vi "Test_KEITHLEY2470.vi"(8 "error in (no error)":errorcluster) -> (0 "error out":errorcluster)   [LabVIEW 2019]
uses:
  Type Definition/handle_Para.ctl
panel:
  in  "VISA resource name out":refnum<visa-resource-name>
  in  "Source Mode  (0: Voltage)":u16(ring) items=["Voltage", "Current"]
  out "lt":u32
  out "Curr[A]":dbl format="%#_6p"
  out "Volt[V]":dbl format="%#_6p"
  in  "STOP":bool
  out "Waveform Chart":cluster{"data[0]":dbl, "data[1]":dbl}(graph)
  in  "READ":bool
  in  "Source Limit Level":dbl=0.01
  in  "Source Level":dbl
  in  "OFF":bool
  in  "ON":bool
  # "KEITHLEY"
  # "2470 SMU"
  # "LEVEL SET"
  # "OUTPUT"
  # "READ"
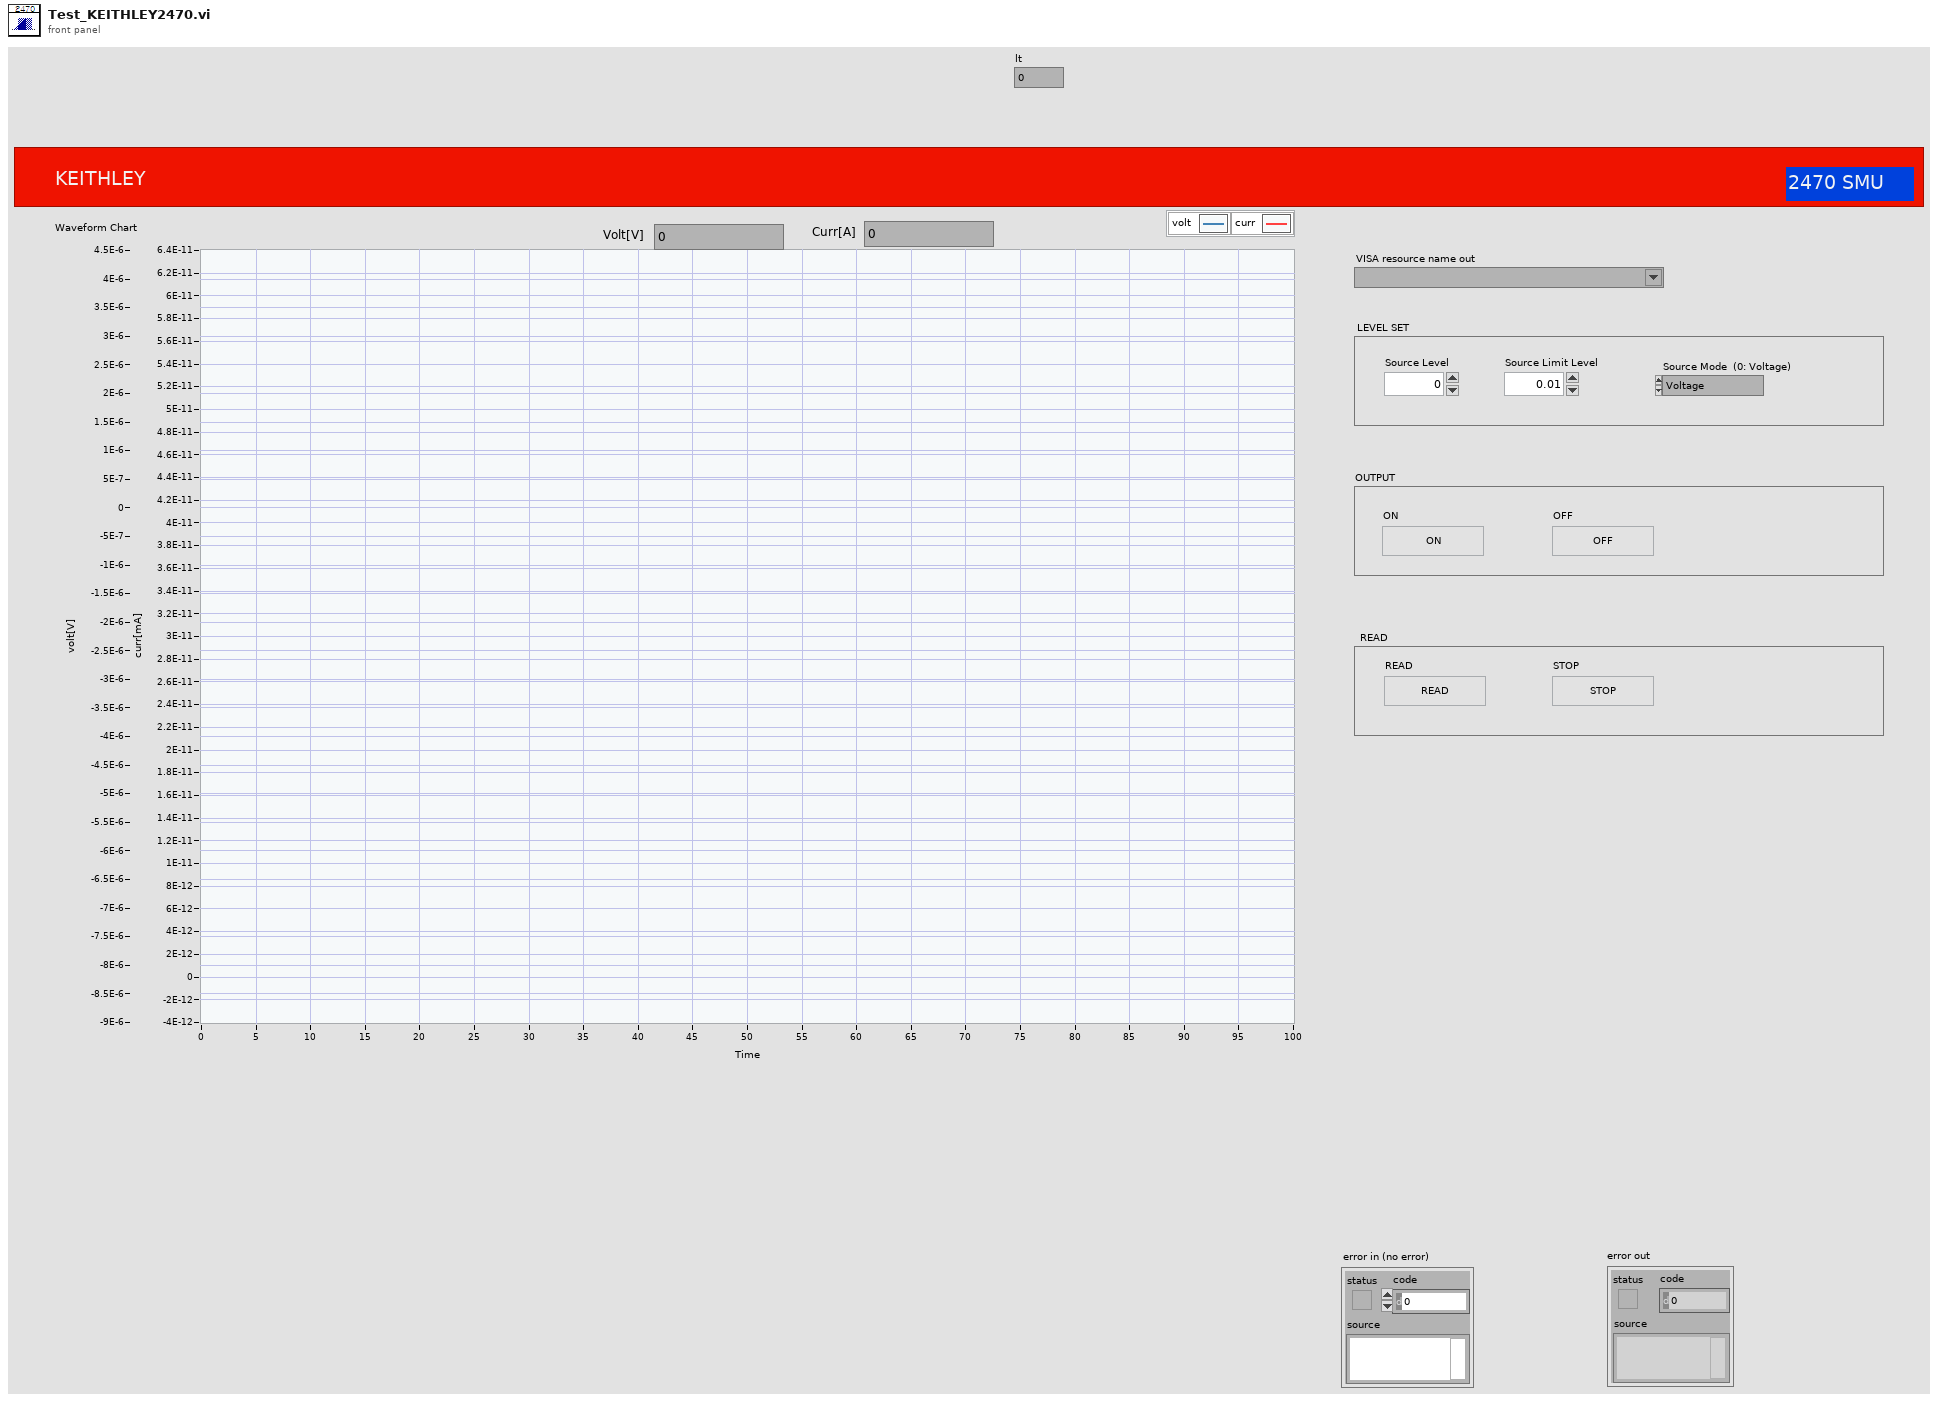
[diagram p1: front panel]
types:
  T1 = typedef "handle_Para.ctl" = cluster{"VISA resource name":refnum<visa-resource-name>, "Function (0: Volts) 1":u16, "Function (0: Volts) 2 ":u16, "Enable Auto Range (T:Enable)":bool, "Source Mode  (0: Voltage)":u16, "Source Level (0)":dbl, "Source Limit Level (0.1)":dbl}
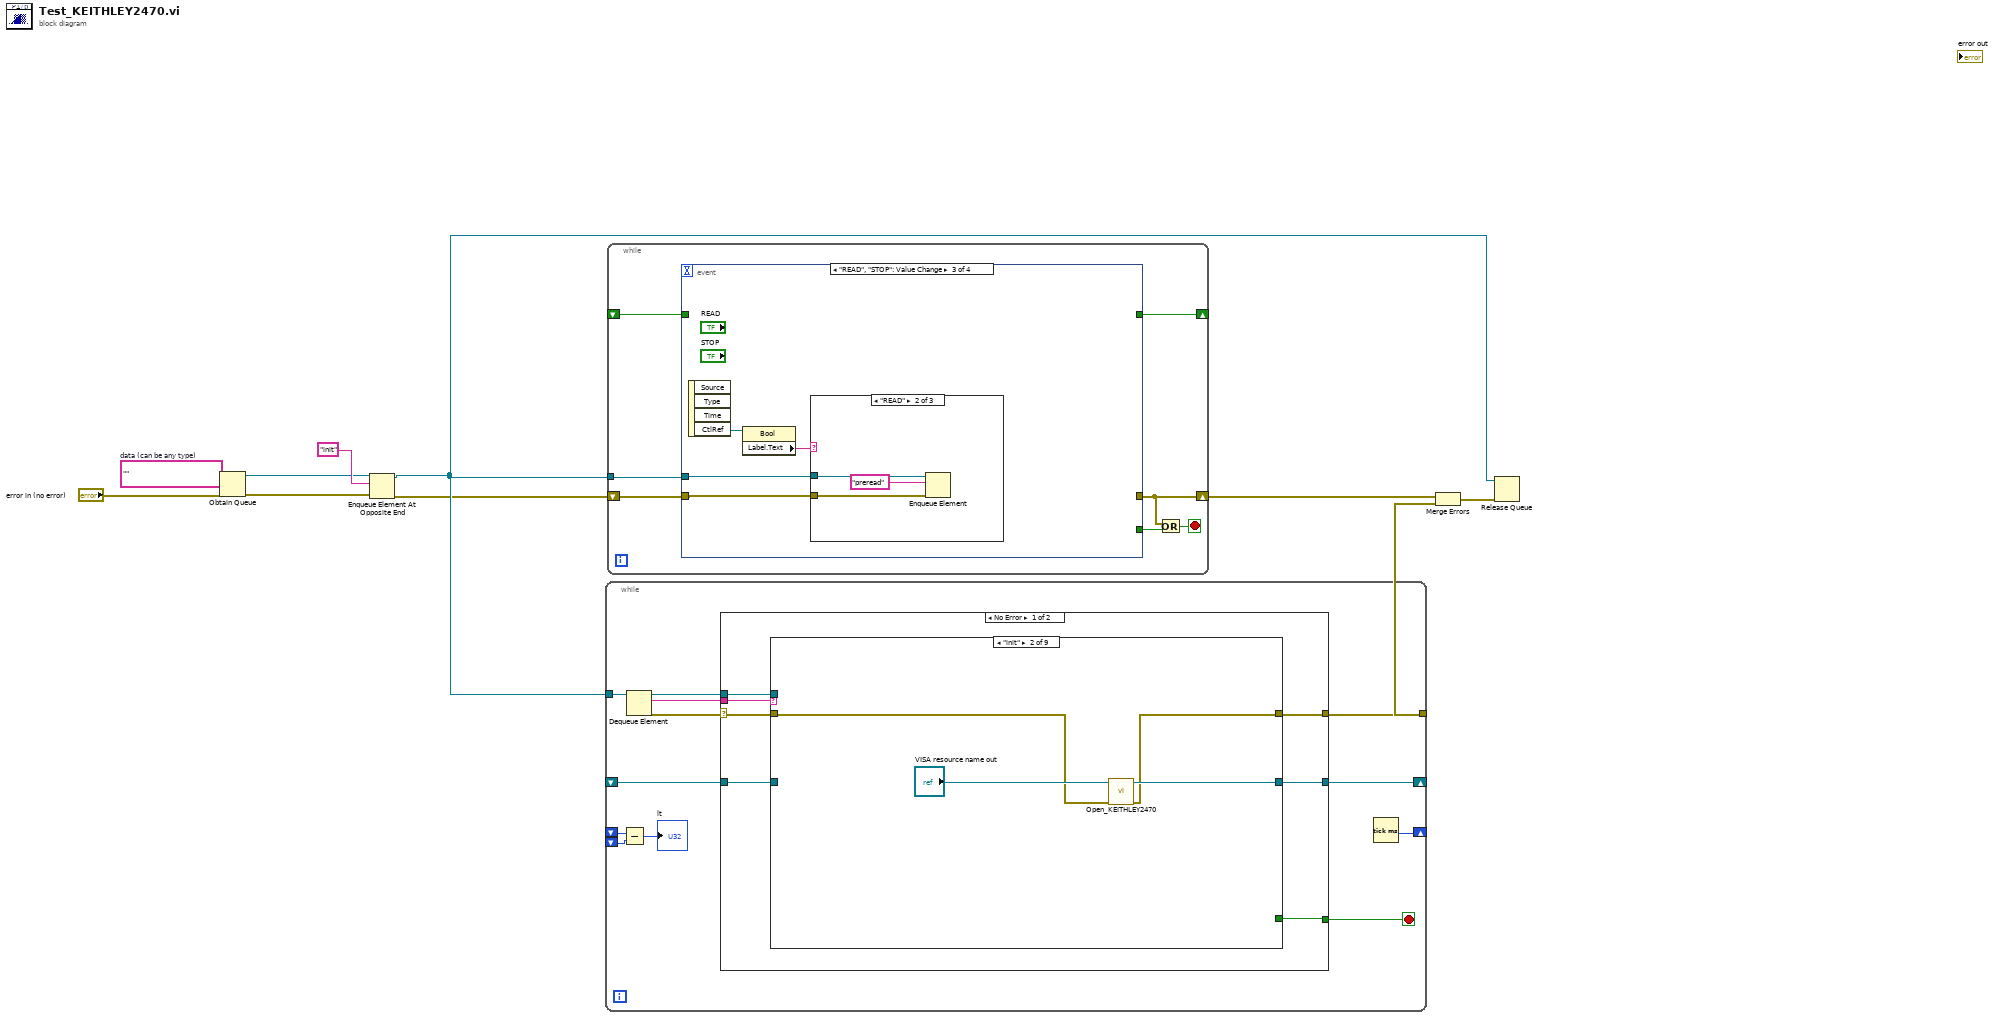
[diagram p0: block diagram]
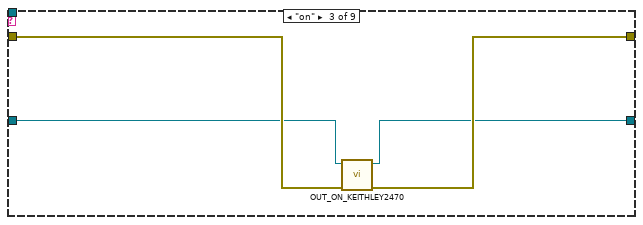
[diagram p3: hidden frame]
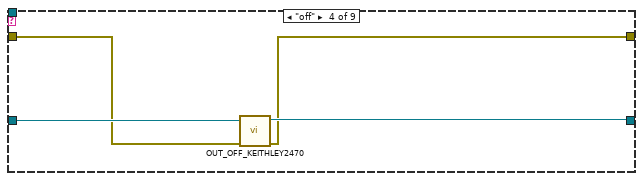
[diagram p4: hidden frame]
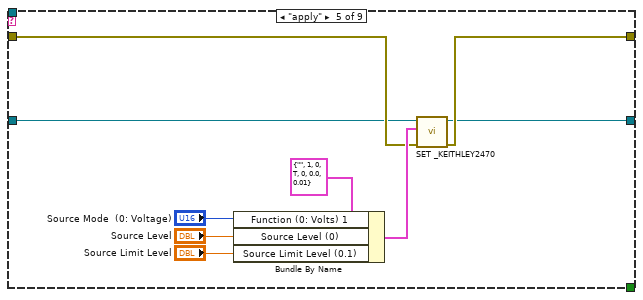
[diagram p5: hidden frame]
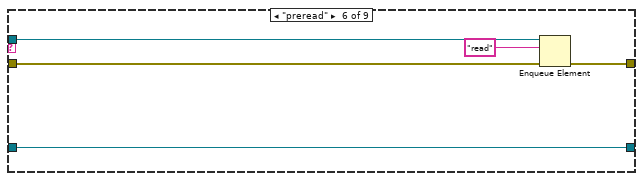
[diagram p6: hidden frame]
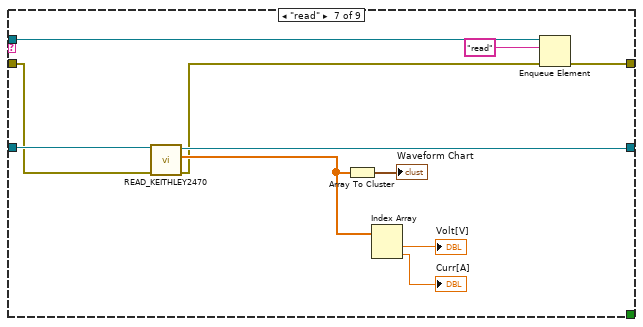
[diagram p7: hidden frame]
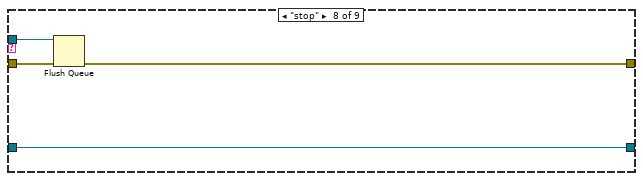
[diagram p8: hidden frame]
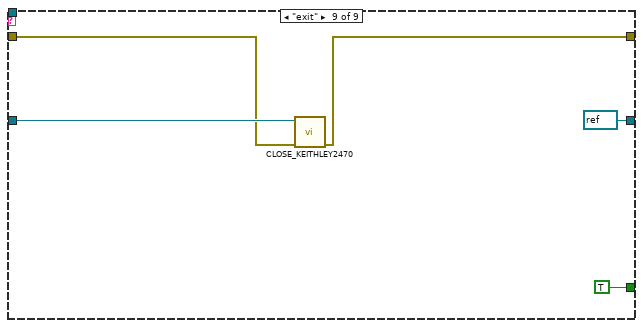
[diagram p9: hidden frame]
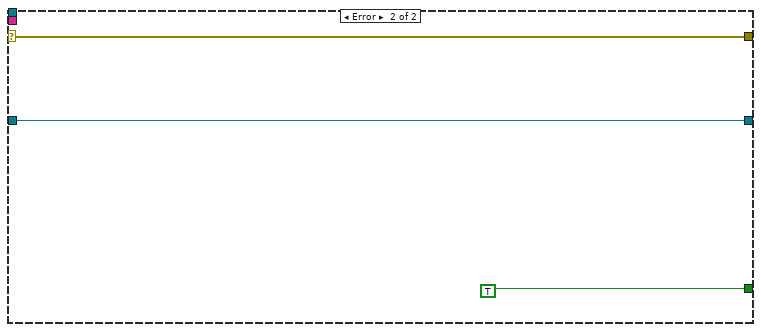
[diagram p10: hidden frame]
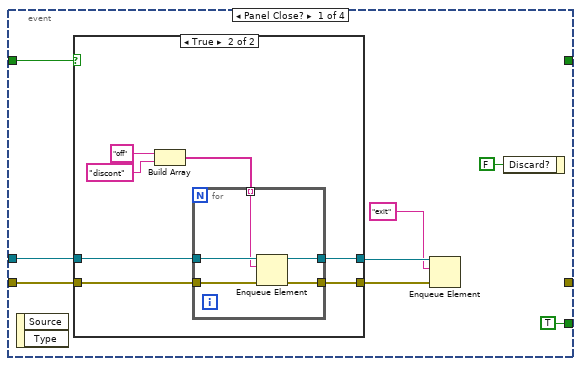
[diagram p11: hidden frame]
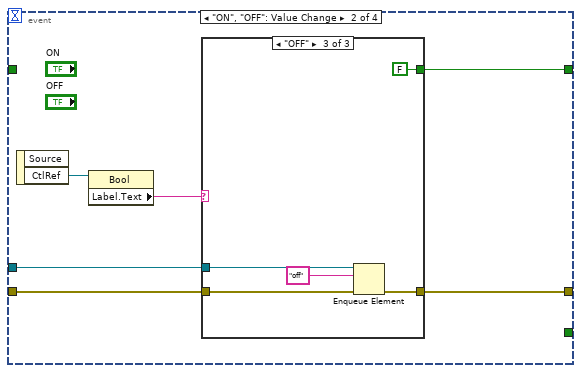
[diagram p13: hidden frame]
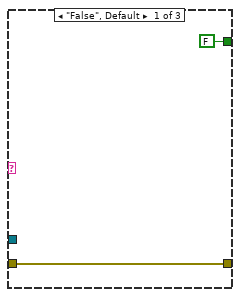
[diagram p14: hidden frame]
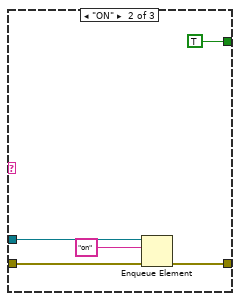
[diagram p15: hidden frame]
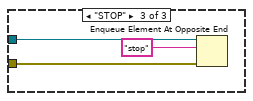
[diagram p17: hidden frame]
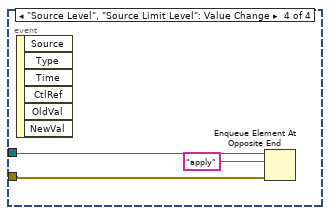
[diagram p18: hidden frame]
diagram:
  w10 = ""  # data (can be any type)
  n1 = Obtain Queue(element data type=w10, error in (no error)="error in (no error)") -> (queue out=w4:refnum<queue>, error out=w2:errorcluster)  [unwired: 3 in, 1 out]
  n2 = Enqueue Element At Opposite End(queue=w4, element="init", error in (no error)=w2) -> (queue out=w3:refnum<queue>, error out=w1:errorcluster)  [unwired: 1 in, 1 out]
  n3 = while {
    tunnel: w3 -> [w22]
    tunnel: [w17] -> w7
    shift-right: [w16] -> _
    shift-left: _ -> [w15]
    shift-left: _ -> [w14]
    shift-right: [w12] -> _
    shift-left: _ -> [w11]
    stop <- w19 stop-if-true
    n4 = Subtract(x=w15, y=w14) -> (x-y=→"lt":u32)
    n5 = Dequeue Element(queue=w22) -> (queue out=w18:refnum<queue>, element=w20:string, error out=w21:errorcluster)  [unwired: 2 in, 1 out]
    n6 = case shown="No Error" w21 {
      selector: w21 -> [w27 w79]
      tunnel: w20 -> [w29 _]
      tunnel: [w26 TRUE] -> w19
      tunnel: w18 -> [w28 _]
      tunnel: [w25 w79] -> w17
      tunnel: [w24 w78] -> w12
      tunnel: w11 -> [w23 w78]
      frame No Error {
        n7 = case shown="\"init\"" w29 {
          tunnel: w28 -> [_ _ _ _ _ w56 w67 w72 _]
          tunnel: w27 -> [w31 w33 w39 w41 w47 w55 w59 w71 w74]
          tunnel: [_ _ _ _ _ _ _ _ TRUE] -> w26
          tunnel: [w31 w32 w38 w40 w46 w54 w63 w69 w73] -> w25
          tunnel: [w30 w34 w36 w42 w44 w53 w60 w70 refnum<visa-resource-name> refnum ("VISA resource name out")] -> w24
          tunnel: w23 -> [w30 _ w37 w43 w45 w53 w61 w70 w76]
          frame "False", Default {
          }
          frame "init" {
            n8 = call "Open_KEITHLEY2470.vi"("error in (no error)"=w33, "KEITHLEY2470"="VISA resource name out") -> ("error out"=w32:errorcluster, "VISA resource name out"=w34:refnum<visa-resource-name>)  [unwired: 8 in]
          }
          frame "on" {
            n9 = call "OUT_ON_KEITHLEY2470.vi"("error in (no error)"=w39, "VISA resource name"=w37) -> ("error out"=w38:errorcluster, "VISA resource name out"=w36:refnum<visa-resource-name>)  [unwired: 8 in]
          }
          frame "off" {
            n10 = call "OUT_OFF_KEITHLEY2470.vi"("error in (no error)"=w41, "VISA resource name"=w43) -> ("error out"=w40:errorcluster, "VISA resource name out"=w42:refnum<visa-resource-name>)  [unwired: 8 in]
          }
          frame "apply" {
            n11 = Bundle By Name(cluster=T1 {"VISA resource name"="", "Function (0: Volts) 1"=1, "Function (0: Volts) 2 "=0, "Enable Auto Range (T:Enable)"=TRUE, "Source Mode  (0: Voltage)"=0, "Source Level (0)"=0.0, "Source Limit Level (0.1)"=0.01} ("Cluster"), "Function (0: Volts) 1"="Source Mode  (0: Voltage)", "Source Level (0)"="Source Level", "Source Limit Level (0.1)"="Source Limit Level") -> (w48:T1)
            n12 = call "SET _KEITHLEY2470.vi"("error in (no error)"=w47, "Cluster"=w48, "VISA resource name"=w45) -> ("error out"=w46:errorcluster, "VISA resource name out"=w44:refnum<visa-resource-name>)  [unwired: 7 in]
          }
          frame "preread" {
            n13 = Enqueue Element(queue=w56, element="read", error in (no error)=w55) -> (error out=w54:errorcluster)  [unwired: 1 in, 2 out]
          }
          frame "read" {
            n14 = call "READ_KEITHLEY2470.vi"("error in (no error)"=w59, "VISA resource name"=w61) -> ("error out"=w58:errorcluster, "DATA"=w62:dbl[], "VISA resource name out"=w60:refnum<visa-resource-name>)  [unwired: 7 in]
            n15 = Array To Cluster(array=w62) -> (cluster=→"Waveform Chart":cluster{"DATA[0]":dbl, "DATA[1]":dbl})
            n16 = Index Array(array=w62) -> (element #1=→"Volt[V]":dbl, element #2=→"Curr[A]":dbl)  [unwired: 2 in]
            n17 = Enqueue Element(queue=w67, element="read", error in (no error)=w58) -> (error out=w63:errorcluster)  [unwired: 1 in, 2 out]
          }
          frame "stop" {
            n18 = Flush Queue(queue=w72, error in (no error)=w71) -> (error out=w69:errorcluster)  [unwired: 2 out]
          }
          frame "exit" {
            n19 = call "CLOSE_KEITHLEY2470.vi"("error in (no error)"=w74, "VISA resource name"=w76) -> ("error out"=w73:errorcluster)  [unwired: 9 in]
          }
        }
      }
      frame Error {
      }
    }
    n20 = Tick Count (ms)() -> (millisecond timer value=w16:u32)
  }
  n21 = while {
    shift-right: [w83] -> w8
    shift-left: w1 -> [w86]
    tunnel: w3 -> [w87]
    shift-right: [w82] -> _
    shift-left: _ -> [w81]
    stop <- w84 stop-if-true
    n22 = event shown="[2] \"READ\", \"STOP\": Value Change" {
      selector: _ -> [_ _ _ _]
      dyn-events: _ -> [_ _ _ _]
      timeout: _ -> [_ _ _ _]
      tunnel: w87 -> [w92 w115 w131 w139]
      tunnel: w86 -> [w91 w114 w130 w138]
      tunnel: [_ w113 _ _] -> w83
      tunnel: [TRUE ("stop") _ _ _] -> w85
      tunnel: [_ w110 _ _] -> w82
      tunnel: w81 -> [w93 _ _ _]
      event Panel Close? {
        n23 = event-data() -> ()  [unwired: 1 in, 2 out]
        n24 = case shown="True" w93 {
          tunnel: w92 -> [w97 w102]
          tunnel: w91 -> [w96 w101]
          tunnel: [w97 w99] -> w90
          tunnel: [w96 w98] -> w89
          frame False {
          }
          frame True {
            n25 = Build Array("off" ("element"), "discont" ("element")) -> (w100:string[])
            n26 = for {
              tunnel: w102 -> [w109]
              tunnel: w101 -> [w108]
              tunnel: w100 -> [w107] mode=indexing
              tunnel: [w106] -> w99
              tunnel: [w105] -> w98
              n27 = Enqueue Element(queue=w109, element=w107, error in (no error)=w108) -> (queue out=w106:refnum<queue>, error out=w105:errorcluster)  [unwired: 1 in, 1 out]
            }
          }
        }
        n28 = Enqueue Element(queue=w90, element="exit", error in (no error)=w89) -> ()  [unwired: 1 in, 3 out]
        n29 = event-data("Discard?"=FALSE) -> ()  [unwired: 1 in, 1 out]
      }
      event "ON", "OFF": Value Change {
        n30 = event-data() -> ("CtlRef"=w112:refnum<vi>)  [unwired: 1 in, 1 out]
        n31 = property class="Bool"(reference=w112) -> ("Label.Text"=w111:string)  [unwired: 1 in, 2 out]
        n32 = case shown="\"OFF\"" w111 {
          tunnel: w115 -> [_ w121 w126]
          tunnel: w114 -> [w117 w120 w125]
          tunnel: [w117 w119 w124] -> w113
          tunnel: [FALSE TRUE FALSE] -> w110
          frame "False", Default {
          }
          frame "ON" {
            n33 = Enqueue Element(queue=w121, element="on", error in (no error)=w120) -> (error out=w119:errorcluster)  [unwired: 1 in, 2 out]
          }
          frame "OFF" {
            n34 = Enqueue Element(queue=w126, element="off", error in (no error)=w125) -> (error out=w124:errorcluster)  [unwired: 1 in, 2 out]
          }
        }
      }
      event "READ", "STOP": Value Change {
        n35 = event-data() -> ("CtlRef"=w129:refnum<vi>)  [unwired: 1 in, 3 out]
        n36 = property class="Bool"(reference=w129) -> ("Label.Text"=w128:string)  [unwired: 1 in, 2 out]
        n37 = case shown="\"READ\"" w128 {
          tunnel: w131 -> [_ w133 w136]
          tunnel: w130 -> [_ w132 w135]
          frame "False", Default {
          }
          frame "READ" {
            n38 = Enqueue Element(queue=w133, element="preread", error in (no error)=w132) -> ()  [unwired: 1 in, 3 out]
          }
          frame "STOP" {
            n39 = Enqueue Element At Opposite End(queue=w136, element="stop", error in (no error)=w135) -> ()  [unwired: 1 in, 3 out]
          }
        }
      }
      event "Source Level", "Source Limit Level": Value Change {
        n40 = event-data() -> ()  [unwired: 1 in, 6 out]
        n41 = Enqueue Element At Opposite End(queue=w139, element="apply", error in (no error)=w138) -> ()  [unwired: 1 in, 3 out]
      }
    }
    n42 = Or(x=w83, y=w85) -> (x .or. y?=w84:bool)
  }
  n43 = Merge Errors(w8, w7) -> (w6:errorcluster)
  n44 = Release Queue(queue=w3, error in (no error)=w6) -> ()  [unwired: 1 in, 3 out]
